vi "Read Frequency.vi"(8 "error in (no error)":errorcluster, 10 "Channel (0: chA)":i32(ring) items=["chA", "chB"], 11 "VISA resource name":refnum<visa-resource-name>) -> (0 "error out":errorcluster, 2 "Frequency":dbl, 3 "VISA resource name out":refnum<visa-resource-name>)   [LabVIEW 2014, in "Stanford Research SR1.lvlib"]
doc: "Reads the frequency of the first waveform in the SR1 Analog Generator."
uses:
  Stanford Research SR1.lvlib
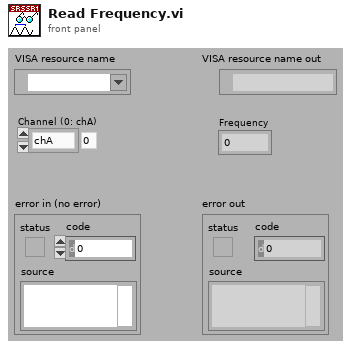
[diagram p1: front panel]
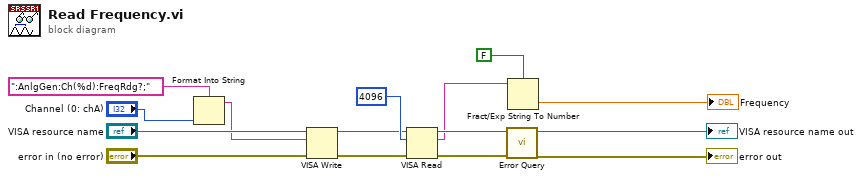
[diagram p0: block diagram]
diagram:
  n1 = Format Into String(format string=":AnlgGen:Ch(%d):FreqRdg?;", "Channel (0: chA)") -> (resulting string=w2:string)  [unwired: 2 in, 1 out]
  n2 = VISA Write(VISA resource name="VISA resource name", write buffer=w2, error in (no error)="error in (no error)") -> (VISA resource name out=w12:refnum<visa-resource-name>, error out=w11:errorcluster)  [unwired: 1 out]
  n3 = VISA Read(VISA resource name=w12, byte count=u32 4096, error in (no error)=w11) -> (VISA resource name out=w10:refnum<visa-resource-name>, read buffer=w5:string, error out=w9:errorcluster)  [unwired: 1 out]
  n4 = call "Error Query.vi"("error in (no error)"=w9, "VISA resource name"=w10) -> ("error out"=→"error out":errorcluster, "VISA resource name out"=→"VISA resource name out":refnum<visa-resource-name>)  [unwired: 6 in, 2 out]
  n5 = Fract/Exp String To Number(use system decimal point (T)=FALSE, string=w5) -> (number=→"Frequency":dbl)  [unwired: 2 in, 1 out]
